vi "Command Header Const.vi"() -> (3 "Command Header":u8[](array[numeric]))   [LabVIEW 2020, in "PicoG-Core.lvlib"]
uses:
  PicoG-Core.lvlib
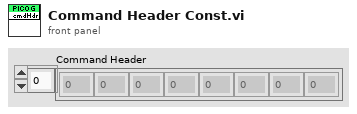
[diagram p1: front panel]
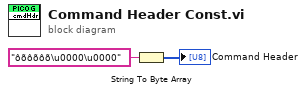
[diagram p0: block diagram]
diagram:
  n1 = String To Byte Array(string="ôõôõôõ\u0000\u0000") -> (unsigned byte array=→"Command Header":u8[])
